vi "DefinidorMissao.vi"(10 "channel":T4) -> (2 "InfoMissao":T1 {"Agentes Disponíveis" format="%#_13g"})   [LabVIEW 2018]
uses:
  <extravilib>/ChannelInstances/Lossy Stream-t'AI Input.ctl'/)Channel.ctl
  Core/AI Input.ctl
  Core/AI Robot.ctl
  Intel/Functions Enum.ctl
  Intel/AttackerStates.ctl
  Path Planning/RRT/PathDests.ctl
  Path Planning/RRT/PathDest.ctl
  Core/AI Ball.ctl
  Core/Field Size.ctl
  Core/AI Judge.ctl
  Intel/Command Enum.ctl
  Util/Events/Events.ctl
  IA Robot Line Display.ctl
  InfoMissao.ctl
  <extravilib>/ChannelInstances/Lossy Stream-t'AI Input.ctl'/Read With Abort.vi
  <extravilib>/ChannelInstances/Lossy Stream-t'AI Input.ctl'/EndpointRead.vi
  <extravilib>/ChannelInstances/Lossy Stream-t'AI Input.ctl'/)Channel.vi
  <resource>/ChannelSupport/_ChannelSupport/WaitIfNeeded.vi
  Util/PreviousState.vi
  <extravilib>/ChannelInstances/Lossy Stream-t'AI Input.ctl'.lvlib
panel:
  in  "id":dbl
  in  "id subs":dbl
  in  "id troca":dbl
  out "Papéis":T2[](array[typedef])
  in  "Troca":bool
  in  "Agentes Disponíveis":dbl format="%#_13g"
  in  "Missões":T5(ring)
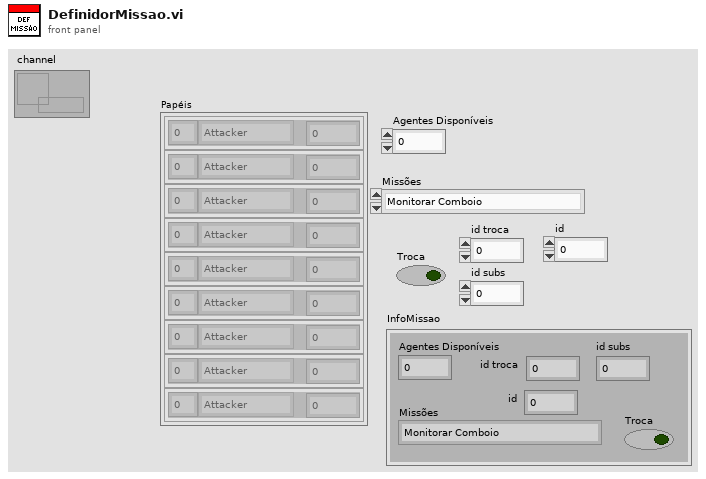
[diagram p1: front panel]
types:
  T1 = typedef "InfoMissao.ctl" = cluster{"Troca ":bool, "Missões ":enum16{"Monitorar Comboio", "Realizar Segurança de Retaguarda", "Vigiar Área", "Reconhecimento de Área"}, "Agentes Disponíveis":dbl, "id troca ":dbl, "id subs":dbl, "id ":dbl}
  T2 = typedef "IA Robot Line Display.ctl" = cluster{"ID":dbl, "function":T3, "number":dbl}
  T3 = typedef "Functions Enum.ctl" = enum16{"None", "Vigia", "2nd Striker", "Attacker", "Goalie", "Defender", "Striker", "Goto 0", "Dummy", "Kicker", "ZigZag 0", "ZigZag 1", "ZigZag 2", "ZigZag 3", "ZigZag 4", "ZigZag 5", "ZigZag 6", "ZigZag 7", "ZigZag 8", ""}
  T4 = typedef "Lossy Stream-t'AI Input.ctl'.lvlib/)Channel.ctl" = refnum<queue>
  T5 = enum16{"Monitorar Comboio", "Realizar Segurança de Retaguarda", "Vigiar Área", "Reconhecimento de Área"}
  T6 = typedef "AI Input.ctl" = cluster{"our_robots":T7[], "enemy_robots":T7[], "balls":T11[], "geometry":T12, "IA Judge":T13, "Received Timestamp":timestamp, "Events":T15}
  T7 = typedef "AI Robot.ctl" = cluster{"id":u32, "function":T3, "x":dbl, "y":dbl, "orientation":dbl, "v_tangent":dbl, "v_normal":dbl, "v_ang":dbl, "kick_x":dbl, "kick_z":dbl, "dribble":bool, "Timestamp":timestamp, "estimatives":cluster{"est_v_tangent":dbl, "est_v_normal":dbl, "est_vx":dbl, "est_vy":dbl, "Pos Robot Est":dbl[]}, "dest_x_kick":dbl, "dest_y_kick":dbl, "Gap Coord":dbl[], "States":T8, "Path ":dbl[][], "Path  Smooth":dbl[][], "Dest":T9, "Missões ":enum16{"Monitorar Comboio", "Realizar Segurança de Retaguarda", "Vigiar Área", "Reconhecimento de Área"}, "Agentes Disponíveis":dbl, "Number":dbl}
  T8 = typedef "AttackerStates.ctl" = enum16{"Pass", "GoToTangent", "BallGetting", "GoToKick", ""}
  T9 = typedef "PathDests.ctl" = T10[]
  T10 = typedef "PathDest.ctl" = cluster{"dest_x":dbl, "dest_y":dbl, "dest_orientation":dbl, "dest_vel":dbl}
  T11 = typedef "AI Ball.ctl" = cluster{"x":dbl, "y":dbl, "timestamp":timestamp, "Vel_x":dbl, "Vel_y":dbl, "Pos Bola Est":dbl[]}
  T12 = typedef "Field Size.ctl" = cluster{"line_width":u32, "field_length":u32, "field_width":u32, "boundary_width":u32, "referee_width":u32, "goal_width":u32, "goal_depth":u32, "goal_wall_width":u32, "center_circle_radius":u32, "defense_radius":u32, "defense_stretch":u32, "free_kick_from_defense_dist":u32, "penalty_spot_from_field_line_dist":u32, "penalty_line_from_spot_dist":u32}
  T13 = typedef "AI Judge.ctl" = cluster{"stage":string, "command":string, "our_goalie_id":dbl, "enemy_goalie_id":dbl, "command enum":T14, "Time":enum16{"Azul", "Amarelo"}}
  T14 = typedef "Command Enum.ctl" = enum16{"Halt", "Stop", "Force Start", "PKA Normal Start", "Prepare Kickoff Ally", "PKE Normal Start", "Prepare Kickoff Enemy", "Prepare Penalty Ally", "PPA Normal Start", "Prepare Penalty Enemy", "PPE Normal Start", "Direct Free Enemy", "Direct Free Ally", "Indirect Free Enemy", "Indirect Free Ally", "Timeout Enemy", "Timeout Ally", "Goal Enemy", "Goal Ally", "Ball Placement Enemy", "Ball Placement Ally", "Normal Half Time", "Extra Time Break", "Extra Half Time", "None", "Post Game"}
  T15 = typedef "Events.ctl" = cluster{"Touch":bool, "Ball out":bool, "id touch":dbl, "Ball out of \nVision":bool, "Ball inside \nGoalie area":bool, "Robot not responding":bool, "Robots responding status":dbl[], "Enemy Ball \nPossession":bool, "Pass State":bool, "id end of pass":dbl, "Kick":bool, "Id ini Possession":dbl, "Ball Possesion":bool, "Id Possesion":dbl, "Direct Kick":bool, "2nd Strk Ativo":bool}
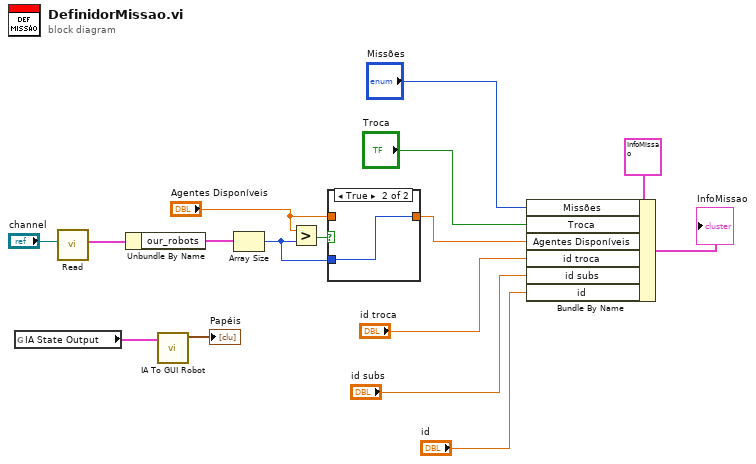
[diagram p0: block diagram]
diagram:
  n1 = global read "PreviousState.vi" "IA State Output"() -> (w10:T6)
  n2 = call <extravilib>:"Read.vi"("channel"="channel") -> ("element"=w11:T6)  [unwired: 5 in, 5 out]
  n3 = Unbundle By Name(w11) -> ("our_robots"=w15:T7[])
  n4 = call "IA To GUI Robot.vi"("Output IA"=w10) -> ("GUI Robot Array"=→"Papéis":T2[])  [unwired: 10 in]
  n5 = Array Size(array=w15) -> (size(s)=w12:i32)
  n6 = Greater?(x="Agentes Disponíveis", y=w12) -> (0:w14:bool)
  n7 = case shown="True" w14 {
    tunnel: [w17 w18] -> w5
    tunnel: "Agentes Disponíveis" -> [w17 _]
    tunnel: w12 -> [_ w18]
    frame False {
    }
    frame True {
    }
  }
  n8 = Bundle By Name(cluster=T1 {"Troca "=FALSE, "Missões "=enum."Monitorar Comboio", "Agentes Disponíveis"=0.0, "id troca "=0.0, "id subs"=0.0, "id "=0.0} ("InfoMissao 2"), "Missões"="Missões", "Troca"="Troca", "Agentes Disponíveis"=w5, "id troca"="id troca", "id subs"="id subs", "id"="id") -> (→"InfoMissao":T1)
